vi "Apply Configurations.vi"(8 "error in (no error)":errorcluster, 11 "Motor in":refnum<class "Motor.lvclass">) -> (0 "error out":errorcluster, 3 "Motor out":refnum<class "Motor.lvclass">)   [LabVIEW 2016, in "Hardware.lvlib" / "Motor.lvlib" / "Motor.lvclass"]
uses:
  <userlib>/Common Components/Hardware/Motor/Motor/Motor.lvclass
  <userlib>/Common Components/Hardware/Motor/Motor/Motor.lvclass/Motor.ctl
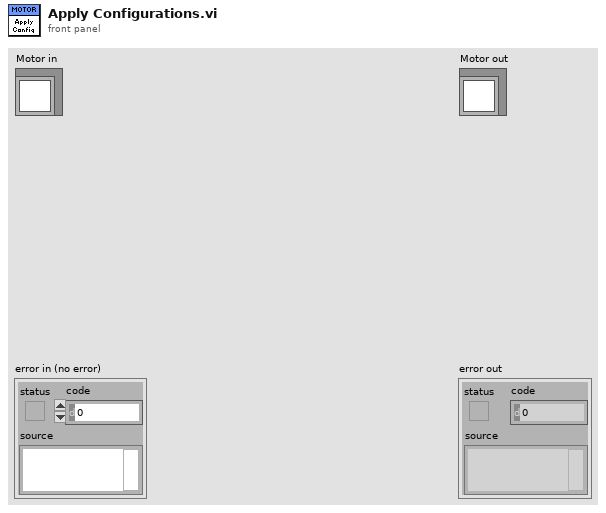
[diagram p1: front panel]
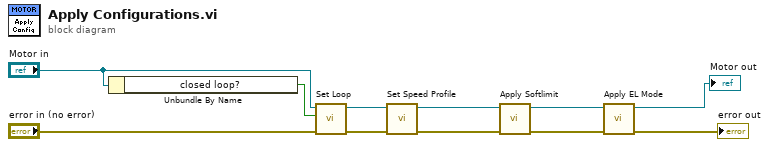
[diagram p0: block diagram]
diagram:
  n1 = Unbundle By Name("Motor in") -> ("closed loop?"=w1:bool)
  n2 = call-dynamic "Set Loop.vi"("error in (no error)"="error in (no error)", "Closed loop?"=w1, "Motor in"="Motor in") -> ("error out"=w4:errorcluster, "Motor out"=w3:refnum<class "Motor.lvclass">)  [unwired: 7 in]
  n3 = call-dynamic "Set Speed Profile.vi"("error in (no error)"=w4, "Motor in"=w3) -> ("error out"=w10:errorcluster, "Motor out"=w8:refnum<class "Motor.lvclass">)  [unwired: 8 in]
  n4 = call <userlib>:"Apply Softlimit.vi"("error in (no error)"=w10, "Motor in"=w8) -> ("error out"=w9:errorcluster, "Motor out"=w6:refnum<class "Motor.lvclass">)  [unwired: 8 in]
  n5 = call <userlib>:"Apply EL Mode.vi"("error in (no error)"=w9, "Motor in"=w6) -> ("error out"=→"error out":errorcluster, "Motor out"=→"Motor out":refnum<class "Motor.lvclass">)  [unwired: 8 in]
